vi "Queue Driver.vi"(0 "States []":string[](array[string]), 5 "Name":string, 11 "Error In":errorcluster, 13 "Operator":T1) -> (4 "Dequeued State":string, 6 "queue out":refnum<queue>, 15 "Error out":errorcluster)   [LabVIEW 2020, in "I2C Controller.lvlib"]
doc: "Able to perform all the queue operation and used move from one state to other."
uses:
  I2C Controller.lvlib
  Typedefs/Operator.ctl
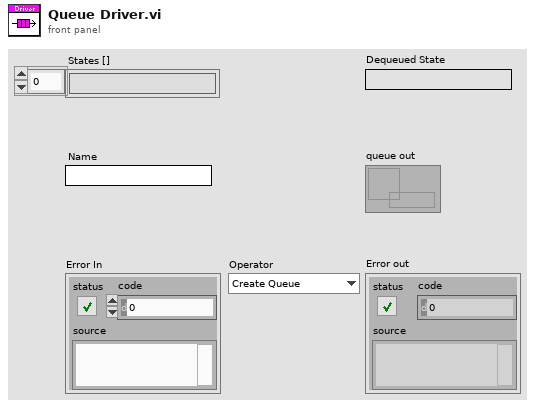
[diagram p1: front panel]
types:
  T1 = typedef "I2C Controller.lvlib/Operator.ctl" = enum16{"Create Queue", "Enqueue", "Enstack", "Dequeue", "Flush Queue", "Release Queue"}
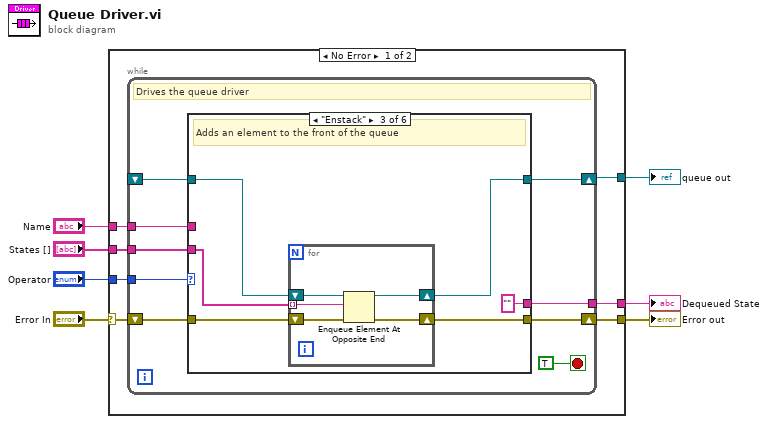
[diagram p0: block diagram]
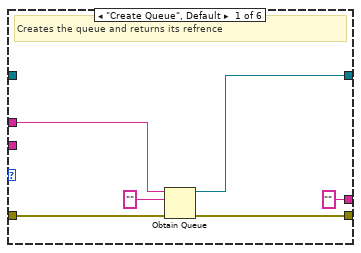
[diagram p2: hidden frame]
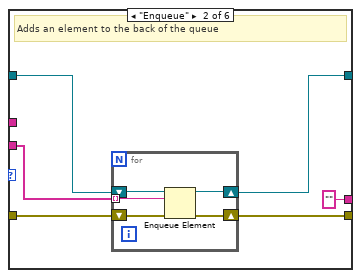
[diagram p3: hidden frame]
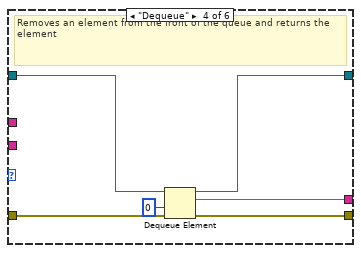
[diagram p4: hidden frame]
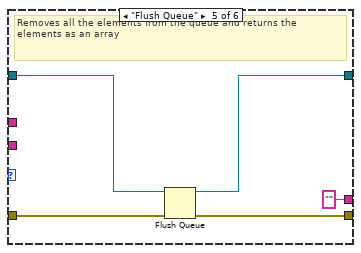
[diagram p5: hidden frame]
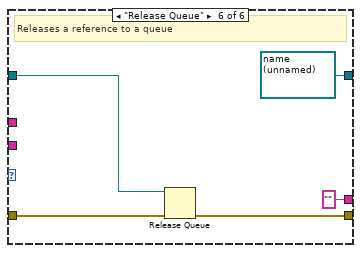
[diagram p6: hidden frame]
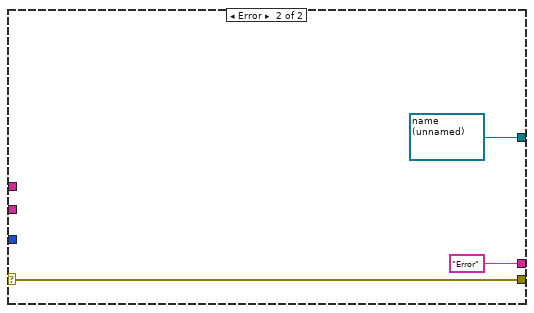
[diagram p7: hidden frame]
diagram:
  n1 = case shown="No Error" "Error In" {
    selector: "Error In" -> [w13 w69]
    tunnel: [w12 w69] -> w6
    tunnel: "Operator" -> [w14 _]
    tunnel: "Name" -> [w11 _]
    tunnel: [w10 refnum<queue> refnum ("queue out")] -> w1
    tunnel: "States []" -> [w9 _]
    tunnel: [w8 "Error" ("name (unnamed)")] -> w2
    frame No Error {
      n2 = while {
        tunnel: w14 -> [w23]
        tunnel: w11 -> [w20]
        shift-right: [w21] -> w12
        shift-left: w13 -> [w22]
        shift-right: [w19] -> w10
        shift-left: _ -> [w18]
        tunnel: w9 -> [w17]
        tunnel: [w16] -> w8
        stop <- TRUE stop-if-true
        # "Drives the queue driver"
        n3 = case shown="\"Enstack\"" w23 {
          tunnel: [w28 w34 w45 w56 w61 w66] -> w21
          tunnel: w22 -> [w29 w35 w46 w57 w62 w67]
          tunnel: w20 -> [w26 _ _ _ _ _]
          tunnel: [w25 w32 w43 w54 w59 refnum<queue> refnum ("queue out")] -> w19
          tunnel: w18 -> [_ w33 w44 w55 w60 w65]
          tunnel: w17 -> [_ w31 w42 _ _ _]
          tunnel: ["" ("name (unnamed)") "" ("name (unnamed)") "" ("name (unnamed)") w53 "" ("name (unnamed)") "" ("name (unnamed)")] -> w16
          frame "Create Queue", Default {
            # "Creates the queue and returns its refrence"
            n4 = Obtain Queue(name (unnamed)=w26, element data type="" ("name (unnamed)"), error in (no error)=w29) -> (queue out=w25:refnum<queue>, error out=w28:errorcluster)  [unwired: 2 in, 1 out]
          }
          frame "Enqueue" {
            # "Adds an element to the back of the queue"
            n5 = for {
              shift-right: [w39] -> w34
              shift-left: w35 -> [w40]
              tunnel: w31 -> [w36] mode=indexing
              shift-right: [w37] -> w32
              shift-left: w33 -> [w38]
              n6 = Enqueue Element(queue=w38, element=w36, error in (no error)=w40) -> (queue out=w37:refnum<queue>, error out=w39:errorcluster)  [unwired: 1 in, 1 out]
            }
          }
          frame "Enstack" {
            # "Adds an element to the front of the queue"
            n7 = for {
              shift-right: [w50] -> w45
              shift-left: w46 -> [w51]
              shift-right: [w48] -> w43
              shift-left: w44 -> [w49]
              tunnel: w42 -> [w47] mode=indexing
              n8 = Enqueue Element At Opposite End(queue=w49, element=w47, error in (no error)=w51) -> (queue out=w48:refnum<queue>, error out=w50:errorcluster)  [unwired: 1 in, 1 out]
            }
          }
          frame "Dequeue" {
            # "Removes an element from the front of the queue and returns the element"
            n9 = Dequeue Element(queue=w55, timeout in ms (-1)=0, error in (no error)=w57) -> (queue out=w54:refnum<queue>, element=w53:string, error out=w56:errorcluster)  [unwired: 1 out]
          }
          frame "Flush Queue" {
            # "Removes all the elements from the queue and returns the elements as an array"
            n10 = Flush Queue(queue=w60, error in (no error)=w62) -> (queue out=w59:refnum<queue>, error out=w61:errorcluster)  [unwired: 1 out]
          }
          frame "Release Queue" {
            # "Releases a reference to a queue"
            n11 = Release Queue(queue=w65, error in (no error)=w67) -> (error out=w66:errorcluster)  [unwired: 1 in, 2 out]
          }
        }
      }
    }
    frame Error {
    }
  }
  "Error out" <- w6
  "Dequeued State" <- w2
  "queue out" <- w1
